vi "AI DAQ.vi"(8 "error in (no error)":errorcluster, 11 "All Queue":T1) -> (0 "error out":errorcluster)   [LabVIEW 2022 SP3]
uses:
  Controls/All Queue Ref.ctl
  Controls/ALL Health.ctl
  <vilib>/Utility/error.llb/DialogType.ctl
  <vilib>/DAQmx/read.llb/DAQmx Read (Analog 1D Wfm NChan NSamp).vi
  6D_Global.vi
  <vilib>/DAQmx/create/scale.llb/DAQmx Create Scale (Map Ranges).vi
  <vilib>/DAQmx/create/channels.llb/DAQmx Create Channel (AI-Voltage-Basic).vi
  <vilib>/DAQmx/configure/timing.llb/DAQmx Timing (Sample Clock).vi
  <vilib>/DAQmx/miscellaneous.llb/DAQmx Fill In Error Info.vi
  <vilib>/measure/madcrms.llb/Averaged DC-RMS for N Chan.vi
  <vilib>/measure/NI_MAPro.lvlib
  <vilib>/DAQmx/configure/trigger.llb/DAQmx Start Trigger (Time).vi
panel:
  # "do confi like this \nVab\ncbc\nvca\nia\nib\nic\nidc\nia_g\nib_g\nic_g\nidc_g\nvab_g\nvbc_g"
  # "Mod 2 - AI7\nAI11\nAI6\nAI12\nAI13\nAI8\nAI9"
  # "Mod 3 AI12\nAI13\nAI8\nAI7\nAI11\nAI10\nAI6\nAI9"
  # "dont mix the config"
  # "Mod3/ai9"
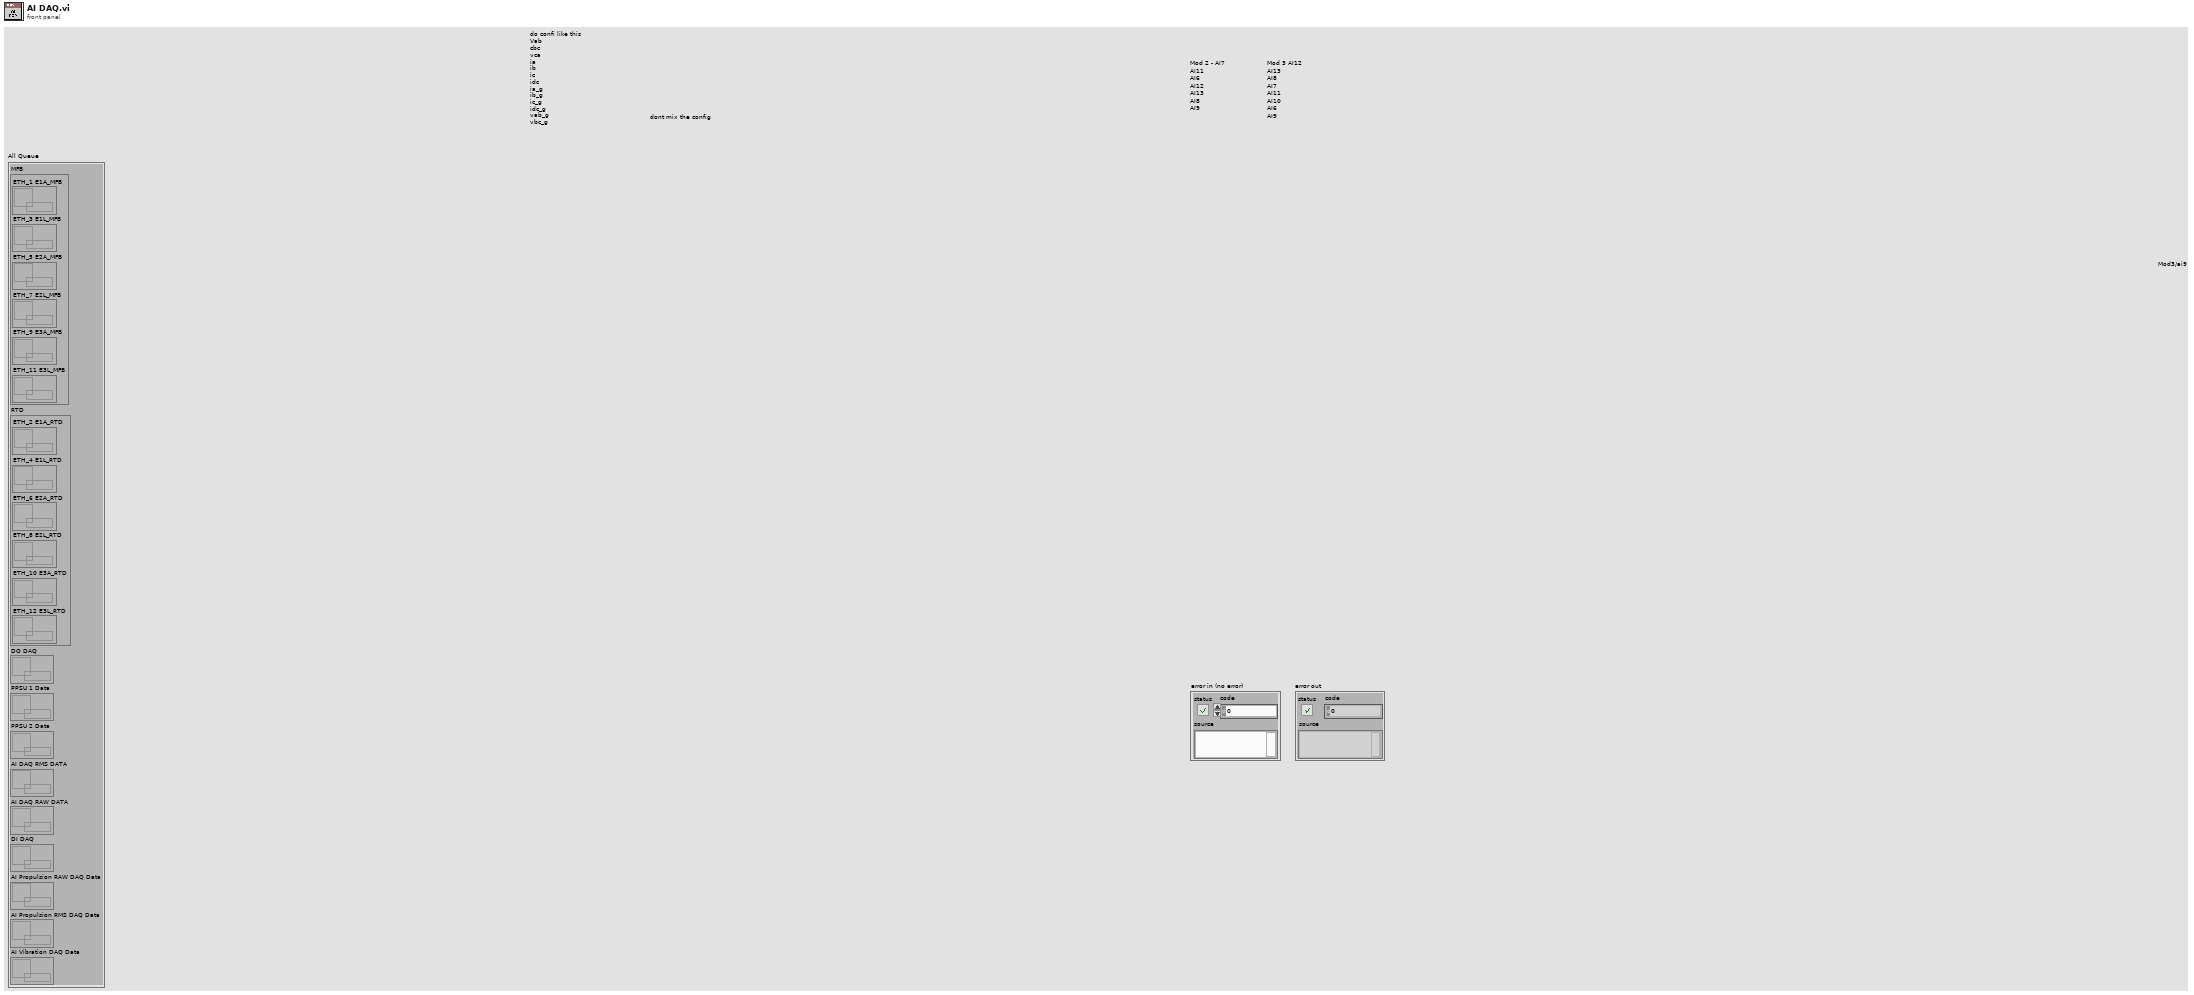
[diagram p1: front panel]
types:
  T1 = typedef "All Queue Ref.ctl" = cluster{"MFB":cluster{"ETH_1 E1A_MFB":refnum<queue>, "ETH_3 E1L_MFB":refnum<queue>, "ETH_5 E2A_MFB":refnum<queue>, "ETH_7 E2L_MFB":refnum<queue>, "ETH_9 E3A_MFB":refnum<queue>, "ETH_11 E3L_MFB":refnum<queue>}, "RTD":cluster{"ETH_2 E1A_RTD ":refnum<queue>, "ETH_4 E1L_RTD ":refnum<queue>, "ETH_6 E2A_RTD ":refnum<queue>, "ETH_8 E2L_RTD ":refnum<queue>, "ETH_10 E3A_RTD ":refnum<queue>, "ETH_12 E3L_RTD ":refnum<queue>}, "DO DAQ":refnum<queue>, "PPSU 1 Data":refnum<queue>, "PPSU 2 Data":refnum<queue>, "AI DAQ RMS DATA":refnum<queue>, "AI DAQ RAW DATA":refnum<queue>, "DI DAQ":refnum<queue>, "AI Propulsion RAW DAQ Data":refnum<queue>, "AI Propulsion RMS DAQ Data":refnum<queue>, "AI Vibration DAQ Data":refnum<queue>}
  T2 = enum16{"Channel Data Input", "Sampling Data Input", "Read Data", "Stop DAQ"}
  T3 = typedef "ALL Health.ctl" = enum16{"AI HS", "AI Vibration HS", "AI Propulsion HS", "DO HS", "Datalog HS", "PPSU HS", "ETH_1 DAQ", "ETH_1 RTD", "ETH_2 DAQ", "ETH_2 RTD", "ETH_5 RTD"}
  T4 = enum16{"Init", "Read 'All'", "Read 'n'", "Read '1'", "Write '1'", "Write 'n'", "Write 'All'"}
  T5 = cluster{"Samples per channel":i32, "Sampling Rate":dbl, "Sample Mode":i32, "Source":tag}
  T6 = cluster{"window for DC":enum16{"Rectangular (none)", "Hanning", "Low side lobe"}, "output function":enum16{"DC only", "RMS only", "DC and RMS"}, "window for RMS":enum16{"Rectangular (none)", "Hanning", "Low side lobe"}, "exp. time constant":dbl, "Ignore input start time":bool}
  T7 = cluster{"AI signal Lists":string, "AI Channel List":tag, "Prescale Min":dbl, "Prescale Max":dbl, "Sensor Min":dbl, "Sensor Max":dbl, "Units":string}[]
  T8 = typedef "DialogType.ctl" = u16
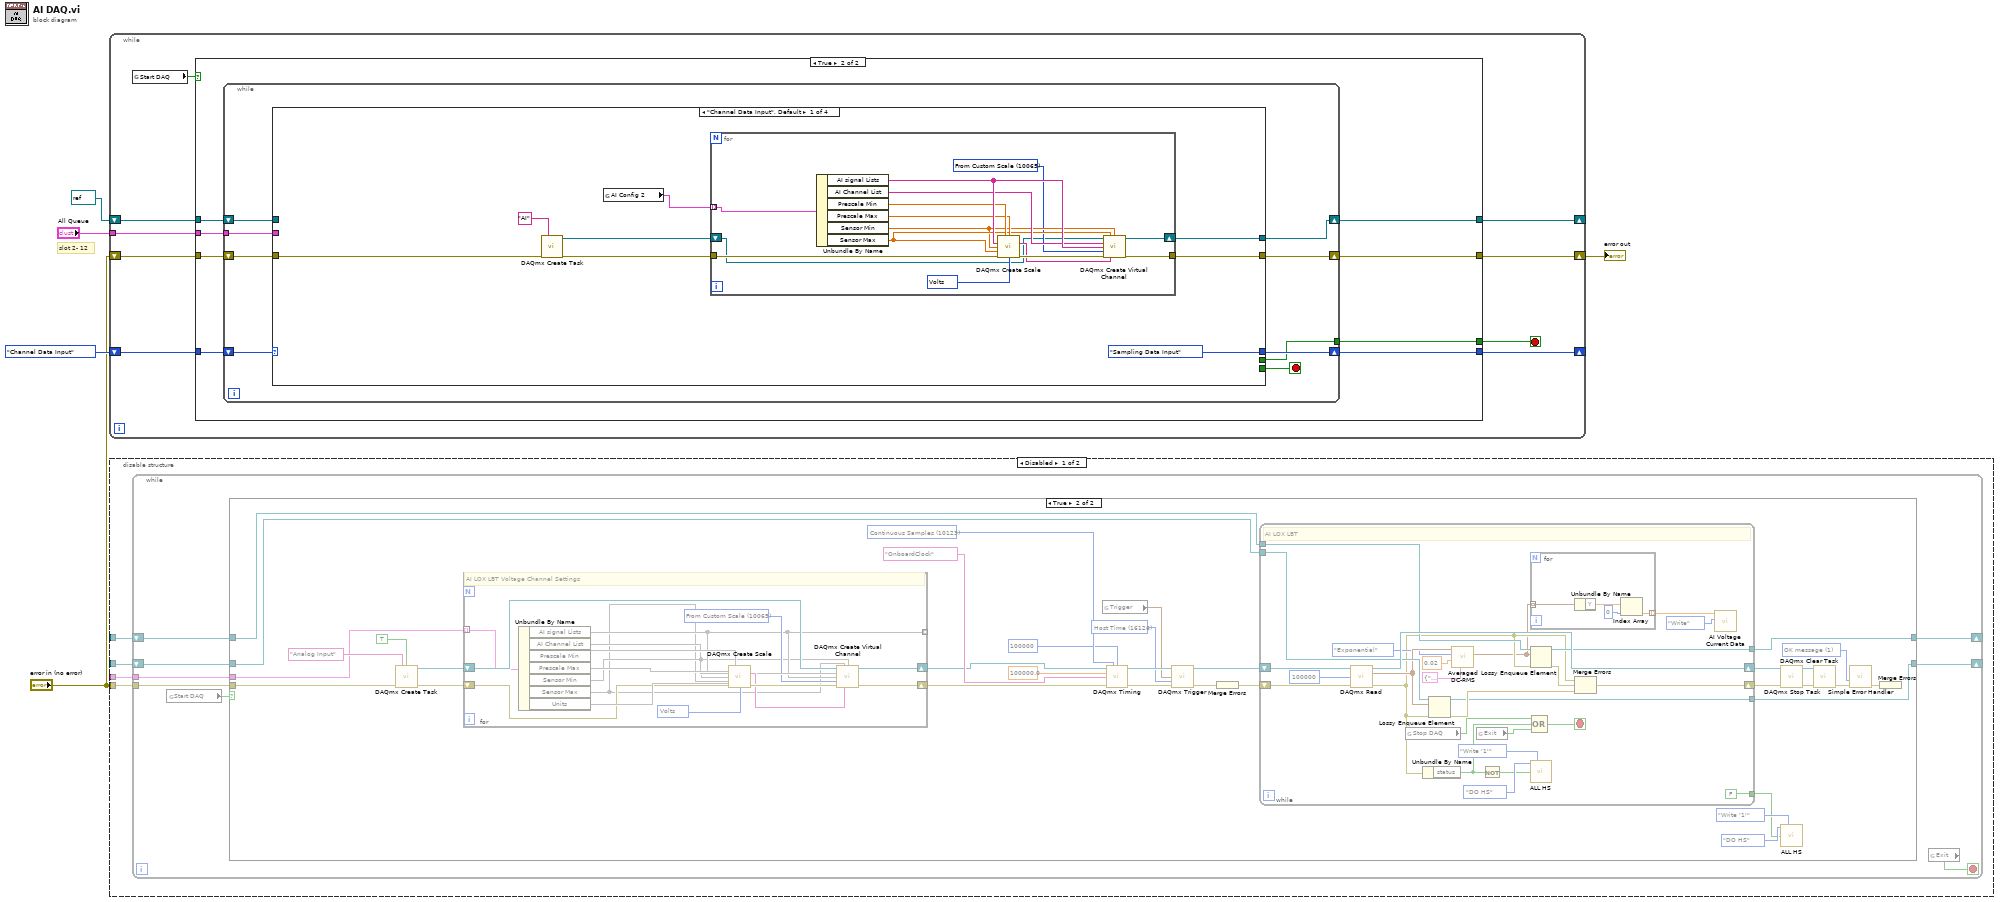
[diagram p0: block diagram]
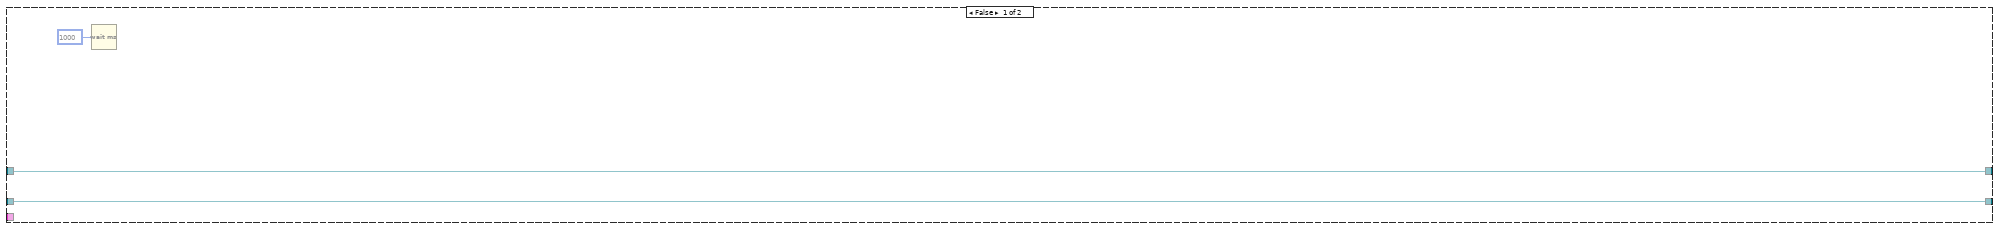
[diagram p2: hidden frame]
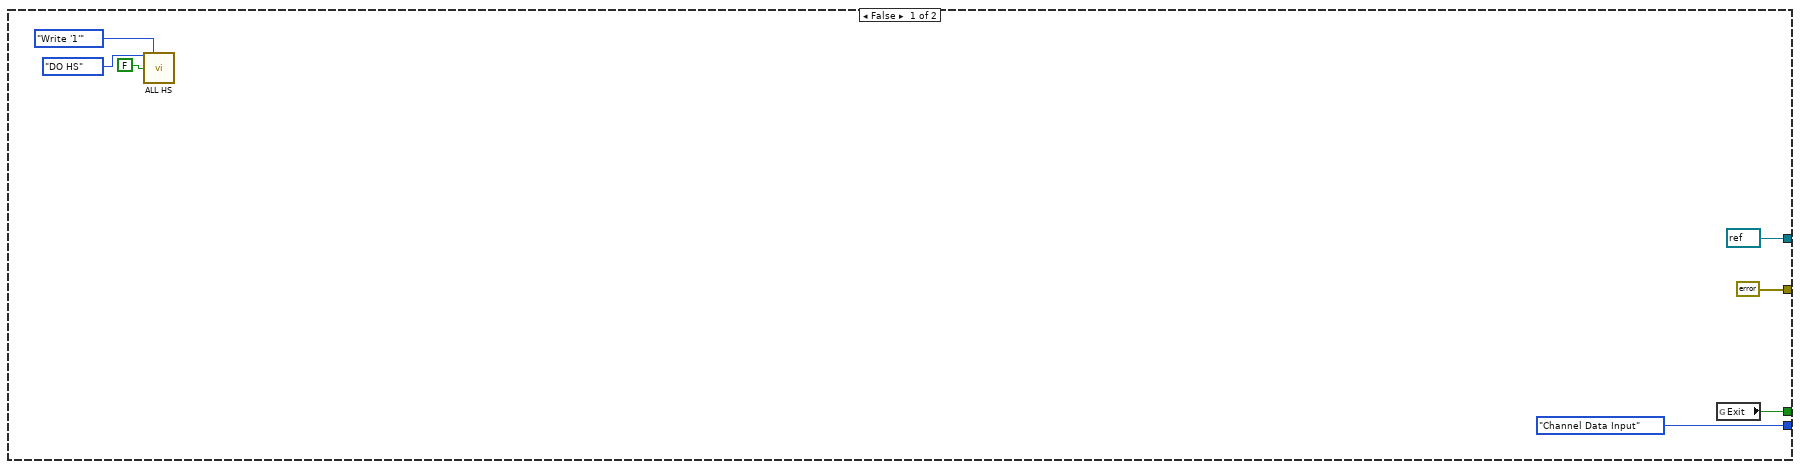
[diagram p4: hidden frame]
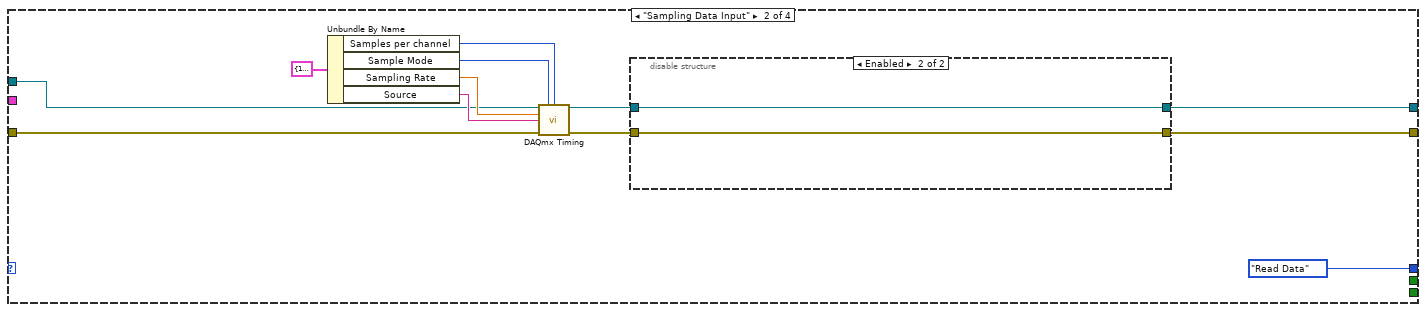
[diagram p5: hidden frame]
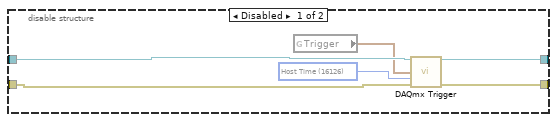
[diagram p6: hidden frame]
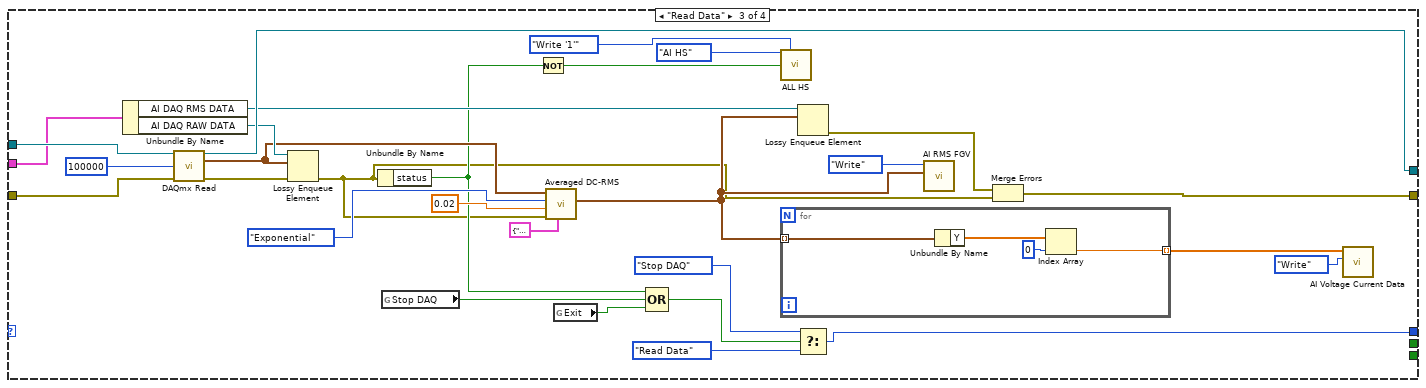
[diagram p7: hidden frame]
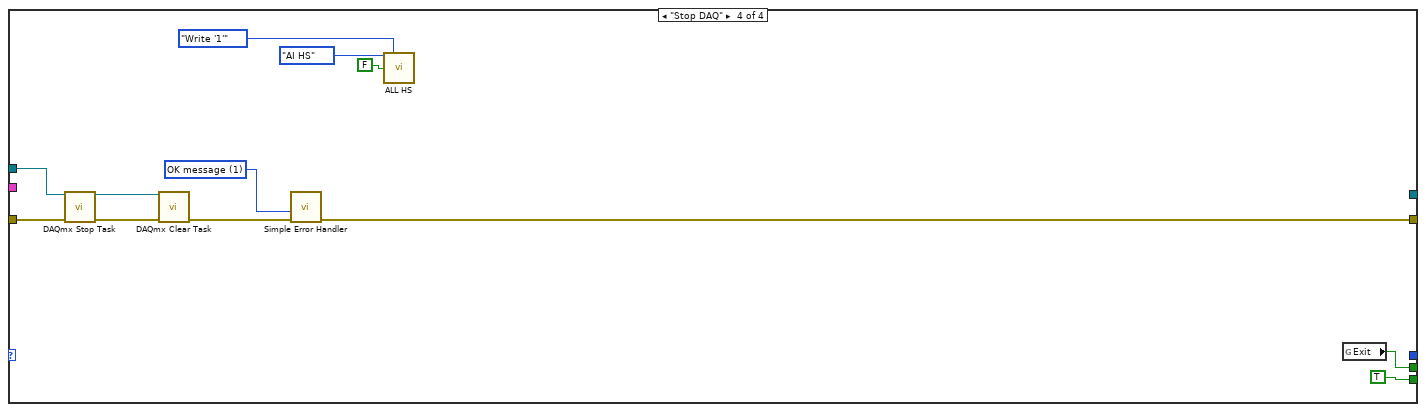
[diagram p8: hidden frame]
diagram:
  # "slot 2- 12"
  n1 = while {
    shift-right: [w11] -> _
    shift-left: T2."Channel Data Input" -> [w14]
    shift-right: [w13] -> _
    shift-left: refnum<k21> refnum ("task out") -> [w12]
    shift-right: [w8] -> w1
    shift-left: "error in (no error)" -> [w9]
    tunnel: "All Queue" -> [w7]
    stop <- w10 stop-if-true
    n2 = global read "6D_Global.vi" "Start DAQ"() -> (w6:bool)
    n3 = case shown="True" w6 {
      tunnel: w14 -> [_ w29]
      tunnel: [refnum<k21> refnum ("task out") w28] -> w13
      tunnel: w12 -> [_ w27]
      tunnel: [T2."Channel Data Input" w26] -> w11
      tunnel: [w19 w25] -> w10
      tunnel: w9 -> [_ w24]
      tunnel: [errorcluster {"status"=FALSE, "code"=0, "source"=""} ("error out") w22] -> w8
      tunnel: w7 -> [_ w23]
      frame False {
        n4 = call "ALL HS.vi"("Loop"=ALL_Health."DO HS", "Option"=T4."Write '1'", "Status"=FALSE) -> ()  [unwired: 10 in, 3 out]
        n5 = global read "6D_Global.vi" "Exit"() -> (w19:bool)
      }
      frame True {
        n6 = while {
          tunnel: [w34] -> w25
          tunnel: w23 -> [w32]
          shift-right: [w35] -> w26
          shift-left: w29 -> [w38]
          shift-right: [w37] -> w28
          shift-left: w27 -> [w36]
          shift-right: [w31] -> w22
          shift-left: w24 -> [w33]
          stop <- w30 stop-if-true
          n7 = case shown="\"Channel Data Input\", Default" w38 {
            tunnel: w33 -> [w40 w67 w105 w126]
            tunnel: [w41 w63 w83 w115] -> w31
            tunnel: [w43 w64 w107 _] -> w37
            tunnel: w36 -> [_ w69 w106 w124]
            tunnel: [T2."Sampling Data Input" T2."Read Data" w108 _] -> w35
            tunnel: [_ _ _ w122] -> w34
            tunnel: w32 -> [_ _ w86 _]
            tunnel: [_ _ _ TRUE] -> w30
            frame "Channel Data Input", Default {
              n8 = call <vilib>:"DAQmx Create Task.vi"("new task name"="AI", "error in"=w40) -> ("task out"=w46:refnum<k21>, "error out"=w45:errorcluster)  [unwired: 12 in]
              n9 = global read "6D_Global.vi" "AI Config 2"() -> (w39:T7)
              n10 = for {
                tunnel: w45 -> [w61]
                tunnel: w39 -> [w59] mode=indexing
                shift-right: [w49] -> w43
                shift-left: w46 -> [w48]
                tunnel: [w47] -> w41
                w50 = 10065 items=["Volts"=10348, "From Custom Scale"=10065] ("units")
                w51 = 10348 items=["Volts"=10348, "Amps"=10342, "Deg F"=10144, "Deg C"=10143, "Deg R"=10145, "Kelvins"=10325, "Strain"=10299, "Ohms"=10384, "Hz"=10373, "Seconds"=10364, "Meters"=10219, "Inches"=10379, "Degrees"=10146, "Radians"=10273, "Ticks"=10304, "g"=10186, "m/s^2"=12470, "m/s"=15959, "in/s"=15960, "Pascals"=10081, "Newtons"=15875, "Pounds"=15876, "kgf"=15877, "psi"=15879, "bar"=15880, "Nm"=15881, "oz-in"=15882, "lb-in"=15883, "lb-ft"=15884, "Volts/Volt"=15896, "mVolts/Volt"=15897, "pCoulombs"=16103, "Coulombs"=16102, "From TEDS"=12516] ("pre-scaled units")
                n11 = Unbundle By Name(w59) -> ("AI signal Lists"=w58:string, "AI Channel List"=w57:tag, "Prescale Min"=w55:dbl, "Prescale Max"=w54:dbl, "Sensor Min"=w52:dbl, "Sensor Max"=w53:dbl)
                n12 = call-poly <vilib>:"DAQmx Create Scale.vi"("pre-scaled minimum"=w55, "pre-scaled maximum"=w54, "name"=w58, "scaled minimum"=w52, "scaled maximum"=w53, "error in"=w61, "pre-scaled units"=w51) -> ("scale out"=w56:tag, "error out"=w60:errorcluster)  [unwired: 7 in]
                n13 = call-poly <vilib>:"DAQmx Create Virtual Channel.vi"("task in"=w48, "maximum value"=w53, "minimum value"=w52, "physical channels"=w57, "name to assign"=w58, "units"=w50, "error in"=w60, "custom scale name"=w56) -> ("task out"=w49:refnum<k21>, "error out"=w47:errorcluster)  [unwired: 6 in]
              }
            }
            frame "Sampling Data Input" {
              n14 = Unbundle By Name(T5 {"Samples per channel"=100000, "Sampling Rate"=100000.0, "Sample Mode"=10123, "Source"="OnboardClock"} ("Analog Input Samples Data")) -> ("Samples per channel"=w70:i32, "Sample Mode"=w71:i32, "Sampling Rate"=w72:dbl, "Source"=w73:tag)
              n15 = call-poly <vilib>:"DAQmx Timing.vi"("task/channels in"=w69, "sample mode"=w71, "samples per channel"=w70, "rate"=w72, "source"=w73, "error in"=w67) -> ("task out"=w66:refnum<k21>, "error out"=w65:errorcluster)  [unwired: 8 in]
              n16 = disable-structure shown="Enabled" {
                disable-tunnel: w66 -> [w79 w81]
                disable-tunnel: w65 -> [w78 w80]
                disable-tunnel: [w77 w81] -> w64
                disable-tunnel: [w76 w80] -> w63
                frame Disabled {
                  w75 = 16126 items=["Host Time"=16126, "I/O Device Time"=16127] ("timescale")
                  n17 = global read "6D_Global.vi" "Trigger"() -> (w74:timestamp)
                  n18 = call-poly <vilib>:"DAQmx Trigger.vi"("task/channels in"=w79, "when"=w74, "timescale"=w75, "error in"=w78) -> ("task out"=w77:refnum<k21>, "error out"=w76:errorcluster)  [unwired: 10 in]
                }
                frame Enabled {
                }
              }
            }
            frame "Read Data" {
              n19 = Unbundle By Name(w86) -> ("AI DAQ RMS DATA"=w101:refnum<queue>, "AI DAQ RAW DATA"=w100:refnum<queue>)
              n20 = call-poly <vilib>:"DAQmx Read.vi"("task/channels in"=w106, "number of samples per channel"=100000, "error in"=w105) -> ("task out"=w107:refnum<k21>, "data"=w99:waveform(dbl)[], "error out"=w85:errorcluster)  [unwired: 10 in]
              n21 = Lossy Enqueue Element(queue=w100, element=w99, error in (no error)=w85) -> (error out=w84:errorcluster)  [unwired: 3 out]
              n22 = Unbundle By Name(w84) -> ("status"=w90:bool)
              n23 = global read "6D_Global.vi" "Stop DAQ"() -> (w94:bool)
              n24 = Not(x=w90) -> (.not. x?=w91:bool)
              n25 = call-poly <vilib>:"Averaged DC-RMS.vi"("averaging control"=T6 {"window for DC"=enum."Rectangular (none)", "output function"=enum."DC and RMS", "window for RMS"=enum."Rectangular (none)", "exp. time constant"=-1.0, "Ignore input start time"=FALSE}, "error in (no error)"=w84, "averaging time"=0.02, "averaging type"=enum16{"Linear", "Exponential"}."Exponential", "signals in"=w99) -> ("RMS value waveforms"=w87:waveform(dbl)[])  [unwired: 2 in, 4 out]
              n26 = global read "6D_Global.vi" "Exit"() -> (w95:bool)
              n27 = Compound Arithmetic op=OR(w90, w94, w95) -> (w89:bool)
              n28 = call "ALL HS.vi"("Loop"=ALL_Health."AI HS", "Option"=T4."Write '1'", "Status"=w91) -> ()  [unwired: 10 in, 3 out]
              n29 = for {
                tunnel: w87 -> [w114] mode=indexing
                tunnel: [w111] -> w98 mode=indexing
                n30 = Unbundle By Name(w114) -> ("Y"=w113:dbl[])
                n31 = Index Array(array=w113, index=0) -> (element=w111:dbl)
              }
              n32 = Lossy Enqueue Element(queue=w101, element=w87) -> (error out=w82:errorcluster)  [unwired: 1 in, 3 out]
              n33 = Select(t=T2."Stop DAQ", s=w89, f=T2."Read Data") -> (s? t:f=w108:T2)
              n34 = call "AI RMS FGV.vi"("RMS value waveforms"=w87, "Enum"=enum16{"Read", "Write"}."Write") -> ()  [unwired: 8 in, 2 out]
              n35 = Merge Errors(w82, w84) -> (w83:errorcluster)
              n36 = call "AI Voltage Current Data.vi"("Enum"=enum16{"Read", "Write"}."Write", "AI Data"=w98) -> ()  [unwired: 8 in, 2 out]
            }
            frame "Stop DAQ" {
              w121 = T8 1 items=["no dialog", "OK message", "continue or stop message", "OK message + warnings", "continue/stop + warnings"] ("type of dialog (OK msg:1)")
              n37 = call <vilib>:"DAQmx Stop Task.vi"("task/channels in"=w124, "error in"=w126) -> ("task out"=w123:refnum<k21>, "error out"=w125:errorcluster)  [unwired: 12 in]
              n38 = call <vilib>:"DAQmx Clear Task.vi"("task in"=w123, "error in"=w125) -> ("error out"=w120:errorcluster)  [unwired: 13 in]
              n39 = call <vilib>:"Simple Error Handler.vi"("type of dialog (OK msg:1)"=w121, "error in (no error)"=w120) -> ("error out"=w115:errorcluster)  [unwired: 3 in, 4 out]
              n40 = call "ALL HS.vi"("Loop"=ALL_Health."AI HS", "Option"=T4."Write '1'", "Status"=FALSE) -> ()  [unwired: 10 in, 3 out]
              n41 = global read "6D_Global.vi" "Exit"() -> (w122:bool)
            }
          }
        }
      }
    }
  }
  "error out" <- w1
  n42 = disable-structure shown="Disabled" {
    disable-tunnel: _ -> [w130 _]
    disable-tunnel: _ -> [w129 _]
    disable-tunnel: "error in (no error)" -> [w128 _]
    disable-tunnel: _ -> [w127 _]
    frame Disabled {
      n43 = while {
        tunnel: w128 -> [w138]
        shift-right: [w137] -> _
        shift-left: w129 -> [w136]
        shift-right: [w134] -> _
        shift-left: w130 -> [w135]
        tunnel: w127 -> [w131]
        stop <- w132 stop-if-true
        n44 = global read "6D_Global.vi" "Start DAQ"() -> (w133:bool)
        n45 = case shown="True" w133 {
          tunnel: w138 -> [_ w153]
          tunnel: [w140 w151] -> w137
          tunnel: w136 -> [w140 w147]
          tunnel: w135 -> [w139 w149]
          tunnel: [w139 w148] -> w134
          tunnel: w131 -> [_ w142]
          frame False {
            n46 = Wait (ms)(milliseconds to wait=u32 1000) -> ()  [unwired: 1 out]
          }
          frame True {
            w156 = 16126 items=["Host Time"=16126, "I/O Device Time"=16127] ("timescale")
            w173 = 10123 items=["Finite Samples"=10178, "Continuous Samples"=10123, "Hardware Timed Single Point"=12522] ("sample mode")
            w167 = T8 1 items=["no dialog", "OK message", "continue or stop message", "OK message + warnings", "continue/stop + warnings"] ("type of dialog (OK msg:1)")
            n47 = call <vilib>:"DAQmx Create Task.vi"("new task name"="Analog Input", "auto cleanup"=TRUE, "error in"=w153) -> ("task out"=w162:refnum<k21>, "error out"=w163:errorcluster)  [unwired: 11 in]
            n48 = for {
              shift-right: [w221] -> w164
              shift-left: w162 -> [w222]
              shift-right: [w219] -> w155
              shift-left: w163 -> [w210]
              tunnel: [w211] -> _ mode=indexing
              tunnel: w142 -> [w207] mode=indexing
              w212 = 10065 items=["Volts"=10348, "From Custom Scale"=10065] ("units")
              w218 = 10348 items=["Volts"=10348, "Amps"=10342, "Deg F"=10144, "Deg C"=10143, "Deg R"=10145, "Kelvins"=10325, "Strain"=10299, "Ohms"=10384, "Hz"=10373, "Seconds"=10364, "Meters"=10219, "Inches"=10379, "Degrees"=10146, "Radians"=10273, "Ticks"=10304, "g"=10186, "m/s^2"=12470, "m/s"=15959, "in/s"=15960, "Pascals"=10081, "Newtons"=15875, "Pounds"=15876, "kgf"=15877, "psi"=15879, "bar"=15880, "Nm"=15881, "oz-in"=15882, "lb-in"=15883, "lb-ft"=15884, "Volts/Volt"=15896, "mVolts/Volt"=15897, "pCoulombs"=16103, "Coulombs"=16102, "From TEDS"=12516] ("pre-scaled units")
              # "AI LOX LBT Voltage Channel Settings"
              n49 = Unbundle By Name(w207) -> ("AI signal Lists"=w211, "AI Channel List"=w213, "Prescale Min"=w215, "Prescale Max"=w214, "Sensor Min"=w209, "Sensor Max"=w208, "Units"=w217)
              n50 = call-poly <vilib>:"DAQmx Create Scale.vi"("pre-scaled minimum"=w215, "pre-scaled maximum"=w214, "name"=w211, "scaled minimum"=w209, "scaled maximum"=w208, "error in"=w210, "pre-scaled units"=w218, "scaled units"=w217) -> ("scale out"=w216:tag, "error out"=w220:errorcluster)  [unwired: 6 in]
              n51 = call-poly <vilib>:"DAQmx Create Virtual Channel.vi"("task in"=w222, "maximum value"=w208, "minimum value"=w209, "physical channels"=w213, "name to assign"=w211, "units"=w212, "error in"=w220, "custom scale name"=w216) -> ("task out"=w221:refnum<k21>, "error out"=w219:errorcluster)  [unwired: 6 in]
            }
            n52 = global read "6D_Global.vi" "Trigger"() -> (w146:timestamp)
            n53 = call-poly <vilib>:"DAQmx Timing.vi"("task/channels in"=w164, "sample mode"=w173, "samples per channel"=100000, "rate"=100000.0, "source"=tag "OnboardClock", "error in"=w155) -> ("task out"=w172:refnum<k21>, "error out"=w158:errorcluster)  [unwired: 8 in]
            n54 = call-poly <vilib>:"DAQmx Trigger.vi"("task/channels in"=w172, "when"=w146, "timescale"=w156, "error in"=w158) -> ("task out"=w159:refnum<k21>, "error out"=w157:errorcluster)  [unwired: 10 in]
            n55 = Merge Errors(w157) -> (w160:errorcluster)
            n56 = while {
              shift-right: [w186] -> w171
              shift-left: w160 -> [w201]
              shift-right: [w200] -> w170
              shift-left: w159 -> [w202]
              tunnel: [w189] -> w151
              tunnel: w147 -> [w194]
              tunnel: w149 -> [w188]
              tunnel: [w187] -> w148
              tunnel: [FALSE ("Status")] -> w143
              i -> [w196]
              stop <- w199 stop-if-true
              # "AI LOX LBT"
              n57 = call-poly <vilib>:"DAQmx Read.vi"("task/channels in"=w202, "number of samples per channel"=100000, "error in"=w201) -> ("task out"=w200:refnum<k21>, "data"=w191:waveform(dbl)[], "error out"=w184:errorcluster)  [unwired: 10 in]
              n58 = global read "6D_Global.vi" "Stop DAQ"() -> (w182:bool)
              n59 = Unbundle By Name(w184) -> ("status"=w198:bool)
              n60 = Lossy Enqueue Element(queue=w194, element=w191, error in (no error)=w184) -> (queue out=w189:refnum<queue>, error out=w197:errorcluster)  [unwired: 2 out]
              n61 = call-poly <vilib>:"Averaged DC-RMS.vi"("averaging control"=T6 {"window for DC"=enum."Rectangular (none)", "output function"=enum."RMS only", "window for RMS"=enum."Rectangular (none)", "exp. time constant"=-1.0, "Ignore input start time"=FALSE}, "averaging time"=0.02, "averaging type"=enum16{"Linear", "Exponential"}."Exponential", "signals in"=w191) -> ("RMS value waveforms"=w183:waveform(dbl)[])  [unwired: 3 in, 4 out]
              n62 = global read "6D_Global.vi" "Exit"() -> (w181:bool)
              n63 = Not(x=w198) -> (.not. x?=w176:bool)
              n64 = for {
                tunnel: w183 -> [w206] mode=indexing
                tunnel: [w204] -> w180 mode=indexing
                n65 = Unbundle By Name ("Get Waveform Components")(w206) -> ("Y"=w205:dbl[])
                n66 = Index Array(array=w205, index=0) -> (element=w204:dbl)
              }
              n67 = Lossy Enqueue Element(queue=w188, element=w183, error in (no error)=w184) -> (queue out=w187:refnum<queue>, error out=w185:errorcluster)  [unwired: 2 out]
              n68 = call "ALL HS.vi"("Loop"=ALL_Health."DO HS", "Option"=T4."Write '1'", "Status"=w176) -> ()  [unwired: 10 in, 3 out]
              n69 = Compound Arithmetic op=OR(w182, w198, w181) -> (w199:bool)
              n70 = Merge Errors(w184, w185, w197) -> (w186:errorcluster)
              n71 = call "AI Voltage Current Data.vi"("Enum"=enum16{"Read", "Write"}."Write", "AI Data"=w180) -> ()  [unwired: 8 in, 2 out]
            }
            n72 = call <vilib>:"DAQmx Stop Task.vi"("task/channels in"=w170, "error in"=w171) -> ("task out"=w165:refnum<k21>, "error out"=w166:errorcluster)  [unwired: 12 in]
            n73 = call "ALL HS.vi"("Loop"=ALL_Health."DO HS", "Option"=T4."Write '1'", "Status"=w143) -> ()  [unwired: 10 in, 3 out]
            n74 = call <vilib>:"DAQmx Clear Task.vi"("task in"=w165, "error in"=w166) -> ("error out"=w152:errorcluster)  [unwired: 13 in]
            n75 = call <vilib>:"Simple Error Handler.vi"("type of dialog (OK msg:1)"=w167, "error in (no error)"=w152) -> ("error out"=w161:errorcluster)  [unwired: 3 in, 4 out]
            n76 = Merge Errors(w161) -> ()  [unwired: 1 out]
          }
        }
        n77 = global read "6D_Global.vi" "Exit"() -> (w132:bool)
      }
    }
    frame Enabled {
    }
  }
